vi "Disonnect from Server.vi"(8 "error in (no error)":errorcluster, 11 "WebSocket Client in":refnum<class "WebSocket Client.lvclass">) -> (0 "error out":errorcluster, 3 "WebSocket Client out":refnum<class "WebSocket Client.lvclass">)   [LabVIEW 2021, in "WebSockets.lvlib" / "WebSocket Client.lvclass"]
doc: "Opens a conenction and creates a new WebSocket Client using the NI VISA TCP Socket.\nWebSockets 2.0.1.40\nSam Sharp - MediaMongrels Ltd\nCopyright (c) 2019, MediaMongrels Ltd"
uses:
  WebSocket Client.lvclass
  C:/my_projects/projects/Algorithms/Labview/21/WebSockets/Source/WebSockets/WebSocket/WebSocket.lvclass
  WebSocket/WebSocket.lvclass/WebSocket.ctl
  WebSocket/Read Socket.vi
  WebSocket/Write Socket.vi
  Sockets/Socket/Socket.lvclass
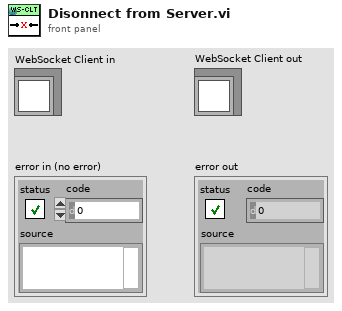
[diagram p1: front panel]
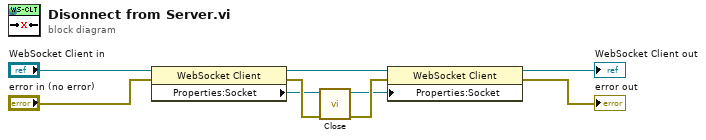
[diagram p0: block diagram]
diagram:
  n1 = property class="WebSocket Client"(reference="WebSocket Client in", error in="error in (no error)") -> (reference out=w7:refnum<class "WebSocket Client.lvclass">, error out=w4:errorcluster, "Properties:Socket"=w1:refnum<class "Socket.lvclass">)
  n2 = call-dynamic "Close.vi"("error in (no error)"=w4, "Socket in"=w1) -> ("error out"=w3:errorcluster, "Socket out"=w2:refnum<class "Socket.lvclass">)  [unwired: 8 in]
  n3 = property class="WebSocket Client"(reference=w7, error in=w3, "Properties:Socket"=w2) -> (reference out=→"WebSocket Client out":refnum<class "WebSocket Client.lvclass">, error out=→"error out":errorcluster)
